vi "digrama_blocos.vi"() -> ()   [LabVIEW 2013]
panel:
  out "A - B":dbl
  out "A +B":dbl
  in  "B":dbl
  in  "A":dbl
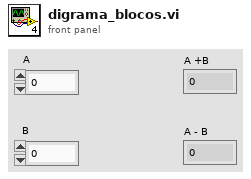
[diagram p1: front panel]
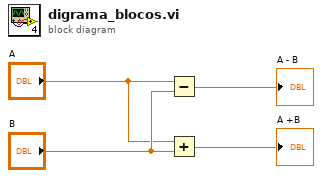
[diagram p0: block diagram]
diagram:
  n1 = Subtract(x="A", y="B") -> (x-y=→"A - B":dbl)
  n2 = Add(x="A", y="B") -> (x+y=→"A +B":dbl)
